vi "FindCase.vi"(1 "Location Tests":T1, 2 "r values":T2 {"r5" format="%.2f"; "r4" format="%.4f"; "r3" format="%.4f"; "r2" format="%.4f"; "r1" format="%.2f"; "r0" format="%.2f"}, 3 "P":cluster{"x":dbl, "y":dbl, "z":dbl}={"x"=1.0, "y"=-5.0, "z"=2.0} {"x" format="%.2f"; "z" format="%.2f"; "y" format="%.2f"}) -> (0 "Case Number":i32)   [LabVIEW 2022 SP3]
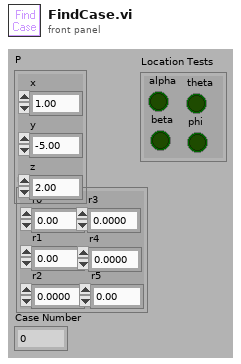
[diagram p1: front panel]
types:
  T1 = cluster{"alpha":bool, "beta":bool, "theta":bool, "phi":bool}
  T2 = cluster{"r0":dbl, "r1":dbl, "r2":dbl, "r3":dbl, "r4":dbl, "r5":dbl}
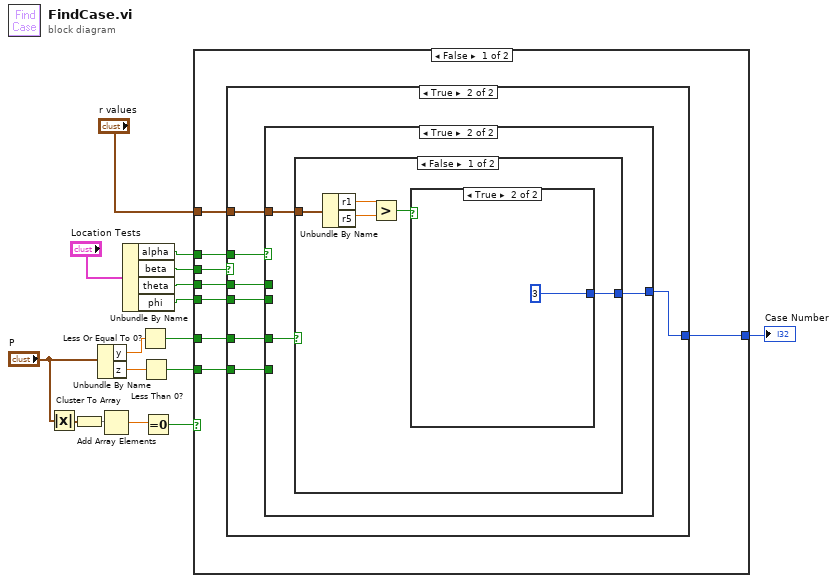
[diagram p0: block diagram]
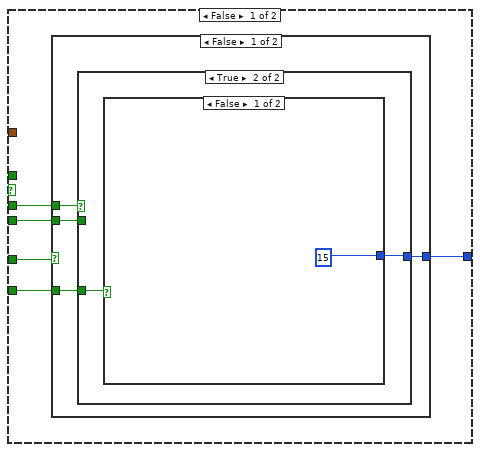
[diagram p2: hidden frame]
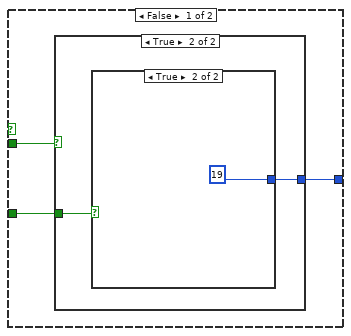
[diagram p3: hidden frame]
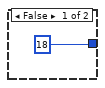
[diagram p4: hidden frame]
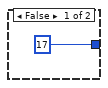
[diagram p5: hidden frame]
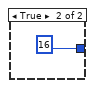
[diagram p6: hidden frame]
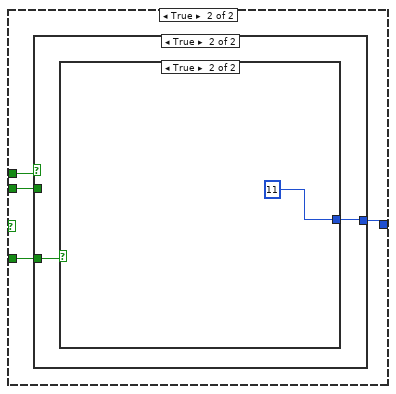
[diagram p7: hidden frame]
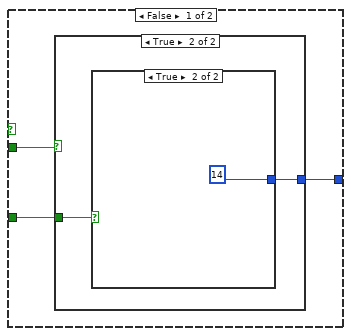
[diagram p8: hidden frame]
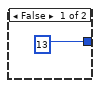
[diagram p9: hidden frame]
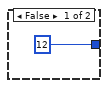
[diagram p10: hidden frame]
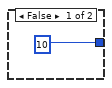
[diagram p11: hidden frame]
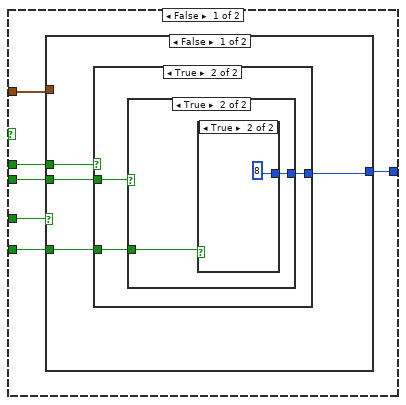
[diagram p12: hidden frame]
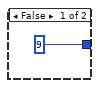
[diagram p13: hidden frame]
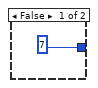
[diagram p14: hidden frame]
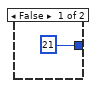
[diagram p15: hidden frame]
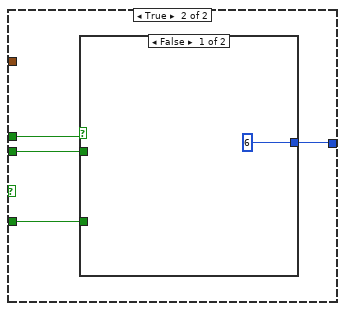
[diagram p16: hidden frame]
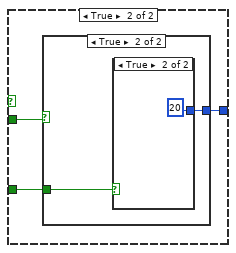
[diagram p17: hidden frame]
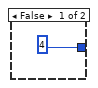
[diagram p18: hidden frame]
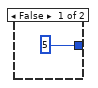
[diagram p19: hidden frame]
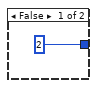
[diagram p20: hidden frame]
diagram:
  n1 = Absolute Value(x="P") -> (abs(x)=w2:cluster{"x":dbl, "y":dbl, "z":dbl})
  n2 = Cluster To Array(cluster=w2) -> (array=w3:dbl[])
  n3 = Unbundle By Name("P") -> ("y"=w10:dbl, "z"=w13:dbl)
  n4 = Add Array Elements(numeric array=w3) -> (sum=w4:dbl)
  n5 = Unbundle By Name("Location Tests") -> ("alpha"=w14:bool, "beta"=w15:bool, "theta"=w8:bool, "phi"=w7:bool)
  n6 = Less Or Equal To 0?(x=w10) -> (x <= 0?=w12:bool)
  n7 = Less Than 0?(x=w13) -> (x < 0?=w9:bool)
  n8 = Equal To 0?(x=w4) -> (x = 0?=w1:bool)
  n9 = case shown="False" w1 {
    tunnel: w15 -> [w24 _]
    tunnel: w14 -> [w23 _]
    tunnel: w12 -> [w22 _]
    tunnel: "r values" -> [w21 _]
    tunnel: w9 -> [w20 _]
    tunnel: w8 -> [w19 _]
    tunnel: w7 -> [w18 _]
    tunnel: [w17 22] -> w6
    frame False {
      n10 = case shown="True" w24 {
        tunnel: w23 -> [_ w68]
        tunnel: w22 -> [w29 w67]
        tunnel: w21 -> [_ w66]
        tunnel: w20 -> [w27 w65]
        tunnel: w19 -> [w28 w63]
        tunnel: w18 -> [w26 w62]
        tunnel: [w25 w64] -> w17
        frame False {
          n11 = case shown="False" w29 {
            tunnel: w28 -> [w33 w49]
            tunnel: w27 -> [w32 w48]
            tunnel: w26 -> [w31 w47]
            tunnel: [w30 w46] -> w25
            frame False {
              n12 = case shown="True" w33 {
                tunnel: [w36 w43] -> w30
                tunnel: w32 -> [w35 w42]
                tunnel: w31 -> [w34 _]
                frame False {
                  n13 = case shown="True" w34 {
                    tunnel: [18 w39] -> w36
                    tunnel: w35 -> [_ w38]
                    frame False {
                    }
                    frame True {
                      n14 = case shown="True" w38 {
                        tunnel: [17 19] -> w39
                        frame False {
                        }
                        frame True {
                        }
                      }
                    }
                  }
                }
                frame True {
                  n15 = case shown="False" w42 {
                    tunnel: [15 16] -> w43
                    frame False {
                    }
                    frame True {
                    }
                  }
                }
              }
            }
            frame True {
              n16 = case shown="True" w49 {
                tunnel: w48 -> [w50 w59]
                tunnel: w47 -> [w51 _]
                tunnel: [w52 w58] -> w46
                frame False {
                  n17 = case shown="True" w51 {
                    tunnel: [13 w55] -> w52
                    tunnel: w50 -> [_ w54]
                    frame False {
                    }
                    frame True {
                      n18 = case shown="True" w54 {
                        tunnel: [12 14] -> w55
                        frame False {
                        }
                        frame True {
                        }
                      }
                    }
                  }
                }
                frame True {
                  n19 = case shown="True" w59 {
                    tunnel: [10 11] -> w58
                    frame False {
                    }
                    frame True {
                    }
                  }
                }
              }
            }
          }
        }
        frame True {
          n20 = case shown="True" w68 {
            tunnel: w67 -> [w74 w103]
            tunnel: w66 -> [w73 w102]
            tunnel: w65 -> [w72 _]
            tunnel: [w71 w101] -> w64
            tunnel: w63 -> [w70 _]
            tunnel: w62 -> [w69 _]
            frame False {
              n21 = case shown="False" w74 {
                tunnel: w73 -> [_ _]
                tunnel: [w78 w91] -> w71
                tunnel: w72 -> [w77 w90]
                tunnel: w70 -> [w75 w88]
                tunnel: w69 -> [w76 w89]
                frame False {
                  n22 = case shown="True" w75 {
                    tunnel: [9 w82] -> w78
                    tunnel: w77 -> [_ w81]
                    tunnel: w76 -> [_ w80]
                    frame False {
                    }
                    frame True {
                      n23 = case shown="True" w80 {
                        tunnel: [7 w85] -> w82
                        tunnel: w81 -> [_ w84]
                        frame False {
                        }
                        frame True {
                          n24 = case shown="True" w84 {
                            tunnel: [21 8] -> w85
                            frame False {
                            }
                            frame True {
                            }
                          }
                        }
                      }
                    }
                  }
                }
                frame True {
                  n25 = case shown="False" w88 {
                    tunnel: [6 w95] -> w91
                    tunnel: w90 -> [_ w94]
                    tunnel: w89 -> [_ w93]
                    frame False {
                    }
                    frame True {
                      n26 = case shown="True" w93 {
                        tunnel: [4 w98] -> w95
                        tunnel: w94 -> [_ w97]
                        frame False {
                        }
                        frame True {
                          n27 = case shown="True" w97 {
                            tunnel: [5 20] -> w98
                            frame False {
                            }
                            frame True {
                            }
                          }
                        }
                      }
                    }
                  }
                }
              }
            }
            frame True {
              n28 = case shown="False" w103 {
                tunnel: w102 -> [w106 w115]
                tunnel: [w104 w111] -> w101
                frame False {
                  n29 = Unbundle By Name(w106) -> ("r1"=w108:dbl, "r5"=w107:dbl)
                  n30 = Greater?(x=w108, y=w107) -> (0:w105:bool)
                  n31 = case shown="True" w105 {
                    tunnel: [2 3] -> w104
                    frame False {
                    }
                    frame True {
                    }
                  }
                }
                frame True {
                  n32 = Unbundle By Name(w115) -> ("r1"=w114:dbl, "r5"=w113:dbl)
                  n33 = Greater?(x=w114, y=w113) -> (0:w112:bool)
                  n34 = case shown="True" w112 {
                    tunnel: [1 0] -> w111
                    frame False {
                    }
                    frame True {
                    }
                  }
                }
              }
            }
          }
        }
      }
    }
    frame True {
      # "test if Point is at origin"
    }
  }
  "Case Number" <- w6
